vi "-8732 Could not replace Attribute--error.vi"(8 "error in":errorcluster, 11 "Attribute":string) -> (0 "error out":errorcluster)   [LabVIEW 2019, in "Config from JSON.lvclass"]
uses:
  Config from JSON.lvclass
  Config from JSON.lvclass/Config from JSON.ctl
  Common-LabVIEW-Helpers/Source/Error Helpers.lvlib
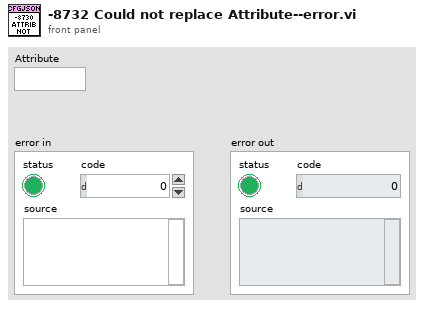
[diagram p1: front panel]
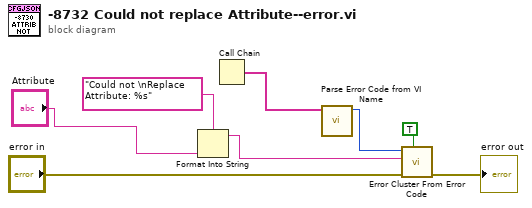
[diagram p0: block diagram]
diagram:
  n1 = Format Into String(format string="Could not \nReplace Attribute: %s" ("error message (\"\")"), "Attribute") -> (resulting string=w6:string)  [unwired: 2 in, 1 out]
  n2 = Call Chain() -> (call chain=w2:string[])
  n3 = call "Parse Error Code from VI Name.vi"("Call Chain"=w2) -> ("Error Code"=w1:i32)  [unwired: 10 in]
  n4 = call <vilib>:"Error Cluster From Error Code.vi"("show call chain? (False)"=TRUE, "error in (no error)"="error in", "error message (\"\")"=w6, "error code (0)"=w1) -> ("error out"=→"error out":errorcluster)  [unwired: 5 in]
